vi "Robot Global Data.vi"() -> ()   [LabVIEW 2012]
doc: "This global VI can contain as many global variables as you need. Place a control on the panel, give it a good name. To read or write to it from a VI, drag the icon to the diagram of that VI. You can also drag from the project. Click on the node to change which global you access. You shouldn't have multiple locations writing to a global or it will cause a race-condition."
uses:
  <vilib>/Rock Robotics/WPI/Camera/WPI_CameraImageSize.ctl
  <vilib>/Rock Robotics/WPI/DriverStation/WPI_DriverStationRobotMode2.ctl
panel:
  in  "Variable Types":T1(tab)
  out "n00bm0d3?":bool
  out "Shift Desired?":bool
  out "High Gear?":bool
  in  "Drive Speed":dbl(knob) scale=-1.0..1.0
  in  "Steering":dbl(knob) scale=-1.0..1.0
  in  "Frisbee Loaded?":bool
  in  "Shooter Speed Control":enum16{"Disable", "Bang-Bang", "PID", "Manual"}(ring)=enum."PID"
  in  "Load Frisbee?":bool
  in  "Manual Shooting?":bool
  in  "Override Shooter?":bool
  in  "Run Shooter?":bool
  in  "Should Fire?":bool
  in  "Shooter Speed Setpoint (Encoder Units)":dbl(slide)=10000.0 scale=0.0..10000.0
  in  "Shooter Speed Reading (Encoder Units)":dbl(knob) scale=0.0..10000.0
  in  "Spatula Down?":bool
  in  "Override Grabbers?":bool
  in  "Reset Lifter?":bool
  in  "Lifter Up?":bool
  out "Tracked Rectangle Y":dbl
  out "Tracked Rectangle X":dbl
  in  "Enable Vision":bool=TRUE
  in  "image size":T2=enum."320x240"
  in  "Requested Auton":string
  in  "Disabled?":bool
  in  "Robot Mode":T3
  in  "LED toggle rate (ms)":u32=20
  out "Autonomous Array":dbl[][](array[numeric])
  # "Each tab contains the global variables that pertain to the different categories."
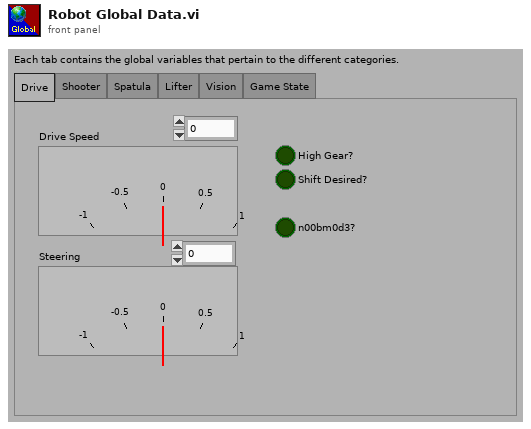
[diagram p1: front panel]
types:
  T1 = enum32{"Drive", "Shooter", "Spatula", "Lifter", "Vision", "Game State"}
  T2 = typedef "WPI_CameraImageSize.ctl" = enum16{"640x480", "320x240", "160x120"}
  T3 = typedef "WPI_DriverStationRobotMode2.ctl" = enum16{"Autonomous Disabled", "Autonomous Enabled", "Teleop Disabled", "Teleop Enabled", "Timeout", "Finish", "Test Disabled", "Test Enabled"}
diagram:
